vi "tsapp_connect_win32.vi"(8 "错误输入（无错误）":errorcluster) -> (0 "错误输出":errorcluster, 1 "tsapp_connect":i32, 2 "ConnectSeccessfully":bool)   [LabVIEW 2016]
uses:
  TSMaster.dll
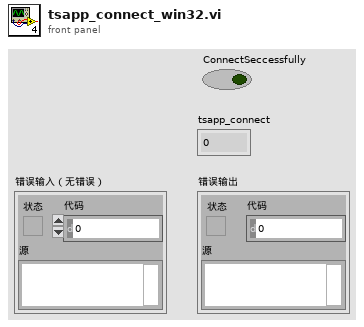
[diagram p1: front panel]
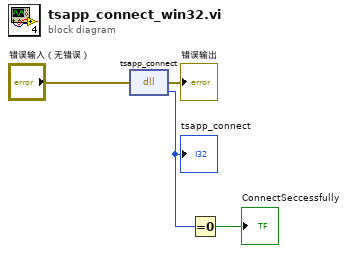
[diagram p0: block diagram]
diagram:
  n1 = dll-call lib="C:/Users/Eric/Desktop/LabVIEW/TSMasterAPI/Win32/CANopen_TS_2015/TSMaster.dll" fn="tsapp_connect"(error in="错误输入（无错误）") -> (error out=→"错误输出":errorcluster, "tsapp_connect"=w2:i32)  [unwired: 2 in, 1 out]
  "tsapp_connect" <- w2
  n2 = Equal To 0?(x=w2) -> (x = 0?=→"ConnectSeccessfully":bool)
